vi "TDMS Release File.vi"(8 "error in (no error)":errorcluster, 11 "Filename":string) -> (0 "error out":errorcluster)   [LabVIEW 2011]
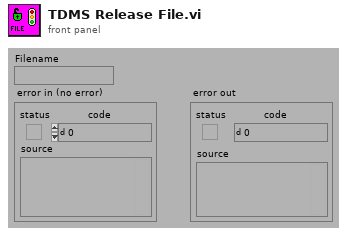
[diagram p1: front panel]
types:
  T1 = typedef "Semaphore RefNum" = refnum<k1>
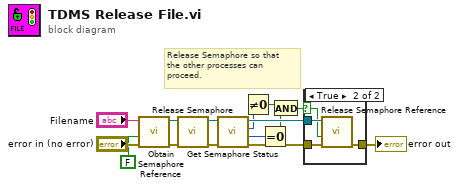
[diagram p0: block diagram]
diagram:
  # "Release Semaphore so that\nthe other processes can\nproceed."
  n1 = call <vilib>:"Obtain Semaphore Reference.vi"("error in (no error)"="error in (no error)", "create if not found (T)"=FALSE, "name (unnamed)"="Filename") -> ("error out"=w12:errorcluster, "semaphore"=w11:T1)  [unwired: 2 in, 1 out]
  n2 = call <vilib>:"Release Semaphore.vi"("error in (no error)"=w12, "semaphore"=w11) -> ("error out"=w10:errorcluster, "semaphore out"=w7:T1)  [unwired: 4 in]
  n3 = call <vilib>:"Get Semaphore Status.vi"("error in (no error)"=w10, "semaphore"=w7) -> ("error out"=w9:errorcluster, "# waiting"=w6:i32, "# available"=w4:i32, "semaphore out"=w8:T1)  [unwired: 4 in, 2 out]
  n4 = Not Equal To 0?(x=w4) -> (x != 0?=w3:bool)
  n5 = Equal To 0?(x=w6) -> (x = 0?=w2:bool)
  n6 = And(x=w3, y=w2) -> (x .and. y?=w1:bool)
  n7 = case shown="True" w1 {
    selector: w1 -> [_ w17]
    tunnel: [w16 w20] -> w14
    tunnel: w9 -> [w16 w19]
    tunnel: w8 -> [_ w18]
    frame False {
    }
    frame True {
      n8 = call <vilib>:"Release Semaphore Reference.vi"("error in (no error)"=w19, "force destroy? (F)"=w17, "semaphore"=w18) -> ("error out"=w20:errorcluster)  [unwired: 7 in, 1 out]
    }
  }
  "error out" <- w14
